vi "Match_Pat_Case_In.vi"(0 "String to match":string, 1 "String":string, 2 "offset (0)":i32) -> (3 "Before Matched string":string, 4 "Matched string":string, 5 "After  Matched string":string, 6 "offset past match":i32)   [LabVIEW 2018]
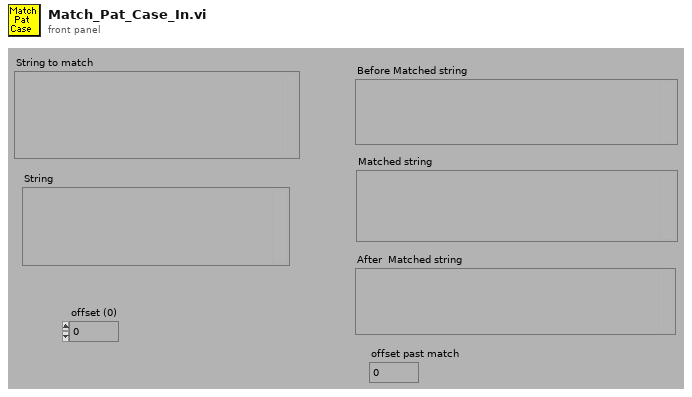
[diagram p1: front panel]
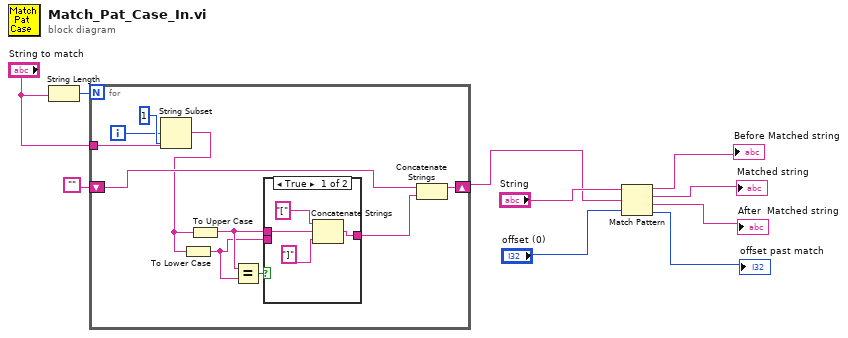
[diagram p0: block diagram]
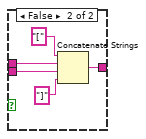
[diagram p2: hidden frame]
diagram:
  n1 = String Length(string="String to match") -> (length=w3:i32)
  n2 = for {
    N: w3 -> [_]
    tunnel: "String to match" -> [w18]
    shift-right: [w16] -> w1
    shift-left: "" -> [w17]
    i -> [w19]
    n3 = String Subset(string=w18, offset (0)=w19, length (rest)=1 ("length")) -> (substring=w14:string)
    n4 = To Lower Case(string=w14) -> (all lower case string=w12:string)
    n5 = To Upper Case(1:w14) -> (0:w13:string)
    n6 = Equal?(x=w13, y=w12) -> (x = y?=w11:bool)
    n7 = case shown="True" w11 {
      tunnel: [w24 w29] -> w15
      tunnel: w13 -> [w23 w28]
      tunnel: w12 -> [_ w27]
      frame True {
        n8 = Concatenate Strings("[", w23, "]" ("Substring")) -> (w24:string)
      }
      frame False {
        n9 = Concatenate Strings("[", w28, w27, "]" ("Substring")) -> (w29:string)
      }
    }
    n10 = Concatenate Strings(w17, w15) -> (w16:string)
  }
  n11 = Match Pattern(string="String", regular expression=w1, offset (0)="offset (0)") -> (before substring=→"Before Matched string":string, match substring=→"Matched string":string, after substring=→"After  Matched string":string, offset past match=→"offset past match":i32)
